vi "Configure Manual Mode Settings.vi"(0 "VISA resource name":refnum<visa-resource-name>, 1 "Memory (1)":i32=1 min=1 max=50 step=1, 5 "Output AC Voltage (115 V)":dbl=115.0 min=0.0 max=300.0 format="%.1f", 7 "Output AC Voltage Frequency (60  Hz)":dbl=60.0 min=45.0 max=500.0 format="%.1p", 9 "Current High Limit (0 A)":dbl min=0.0 max=36.8 format="%.3f", 11 "error in (no error)":errorcluster, 12 "Voltage Range Mode (1:Auto)":u16(ring)=1 items=["High", "Auto"]) -> (4 "VISA resource name out":refnum<visa-resource-name>, 15 "error out":errorcluster)   [LabVIEW 2020, in "eec 6700.lvlib"]
doc: "Configures the manual mode settings to the power source instrument."
uses:
  <instrlib>/EEC6700LV-driver/eec 6700.lvlib
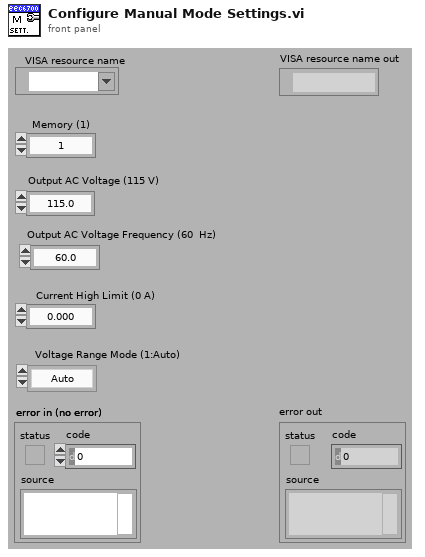
[diagram p1: front panel]
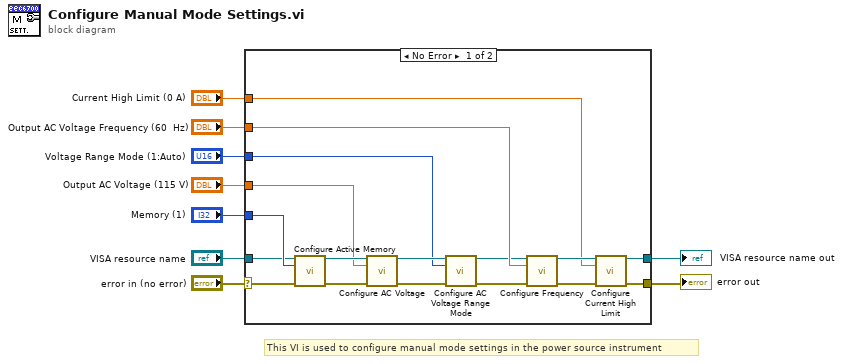
[diagram p0: block diagram]
diagram:
  # "This VI is used to configure manual mode settings in the power source instrument"
  n1 = case shown="No Error" "error in (no error)" {
    selector: "error in (no error)" -> [w15 w28]
    tunnel: "VISA resource name" -> [w16 w27]
    tunnel: [w19 w27] -> w8
    tunnel: [w20 w28] -> w7
    tunnel: "Memory (1)" -> [w24 _]
    tunnel: "Output AC Voltage (115 V)" -> [w17 _]
    tunnel: "Output AC Voltage Frequency (60  Hz)" -> [w23 _]
    tunnel: "Current High Limit (0 A)" -> [w18 _]
    tunnel: "Voltage Range Mode (1:Auto)" -> [w10 _]
    frame No Error {
      n2 = call <instrlib>:"Configure Active Memory.vi"("VISA resource name"=w16, "Memory (1)"=w24, "error in (no error)"=w15) -> ("VISA resource name out"=w25:refnum<visa-resource-name>, "error out"=w26:errorcluster)  [unwired: 11 in]
      n3 = call <instrlib>:"Configure AC Voltage.vi"("VISA resource name"=w25, "Output AC Voltage (115 V)"=w17, "error in (no error)"=w26) -> ("VISA resource name out"=w14:refnum<visa-resource-name>, "error out"=w12:errorcluster)  [unwired: 11 in]
      n4 = call <instrlib>:"Configure AC Voltage Range Mode.vi"("VISA resource name"=w14, "Voltage Range Mode (1:Auto)"=w10, "error in (no error)"=w12) -> ("VISA resource name out"=w13:refnum<visa-resource-name>, "error out"=w11:errorcluster)  [unwired: 11 in]
      n5 = call <instrlib>:"Configure Frequency.vi"("VISA resource name"=w13, "Output AC Voltage Frequency (60  Hz)"=w23, "error in (no error)"=w11) -> ("VISA resource name out"=w22:refnum<visa-resource-name>, "error out"=w21:errorcluster)  [unwired: 11 in]
      n6 = call <instrlib>:"Configure Current High Limit.vi"("VISA resource name"=w22, "Current High Limit (0 A)"=w18, "error in (no error)"=w21) -> ("VISA resource name out"=w19:refnum<visa-resource-name>, "error out"=w20:errorcluster)  [unwired: 11 in]
    }
    frame Error {
    }
  }
  "error out" <- w7
  "VISA resource name out" <- w8
